vi "Index Created for lvproj.vi"(8 "error in (no error)":errorcluster, 11 "Indexing Test Finder Test in":refnum<class "Indexing Test Finder Test.lvclass">) -> (0 "error out":errorcluster, 3 "Indexing Test Finder Test out":refnum<class "Indexing Test Finder Test.lvclass">)   [LabVIEW 2020, in "LUnit Tests.lvlib" / "Indexing Test Finder Test.lvclass"]
uses:
  Indexing Test Finder Test.lvclass
  Indexing Test Finder Test.lvclass/Indexing Test Finder Test.ctl
  source/Framework/Helper Classes/Test Finder/Test Finder.lvclass
  Test Finder/Finder Test.lvclass
  c59a45e6-8387-4d73-9fe8-839093b27eb6.vi
  <vilib>/Astemes/LUnit/Test Case.lvclass
  C:/Git/astemes-lunit/tests/Test Finder/Finder Test.lvclass
  C:/Program Files (x86)/National Instruments/LabVIEW 2020/vi.lib/Astemes/LUnit/Test Case.lvclass
  C:/Git/astemes-lunit/tests/Indexing Test Finder Test/Indexing Test Finder Test.lvclass
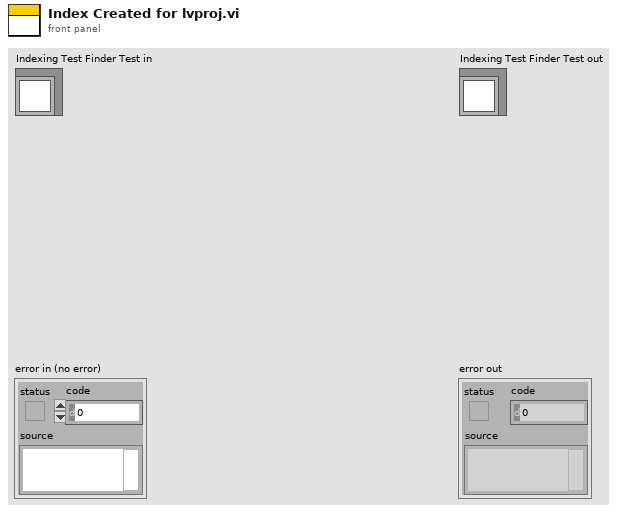
[diagram p1: front panel]
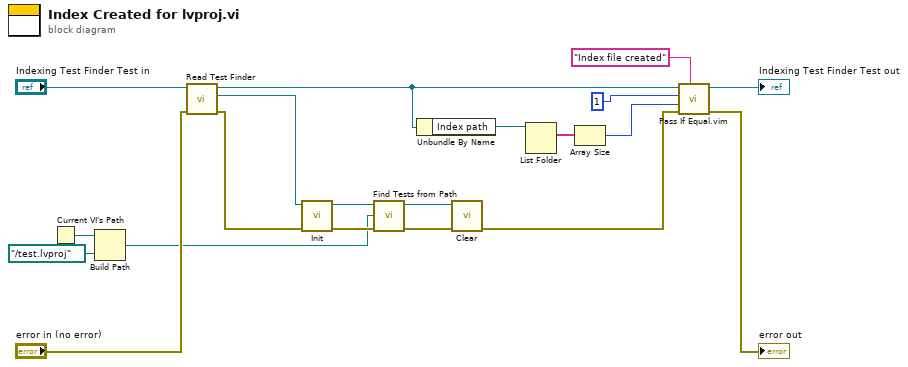
[diagram p0: block diagram]
diagram:
  n1 = Current VI's Path() -> (path=w12:path)
  n2 = Build Path(base path=w12, name or relative path=path "../test.lvproj") -> (appended path=w10:path)
  n3 = call "Read Test Finder.vi"("error in (no error)"="error in (no error)", "Test Finder In"="Indexing Test Finder Test in") -> ("error out"=w14:errorcluster, "Test Finder.lvclass"=w15:refnum<class "Test Finder.lvclass">, "Test Finder Out"=w4:refnum<class "Indexing Test Finder Test.lvclass">)  [unwired: 7 in]
  n4 = call-dynamic "Init.vi"("error in (no error)"=w14, "Test Finder in"=w15) -> ("error out"=w18:errorcluster, "Test Finder out"=w19:refnum<class "Test Finder.lvclass">)  [unwired: 8 in]
  n5 = call-dynamic "Find Tests from Path.vi"("error in (no error)"=w18, "Project or Class Path"=w10, "Test Case Finder In"=w19) -> ("error out"=w16:errorcluster, "Test Case Finder Out"=w17:refnum<class "Test Finder.lvclass">)  [unwired: 7 in]
  n6 = Unbundle By Name(w4) -> ("Index path"=w8:path)
  n7 = call "Clear.vi"("error in (no error)"=w16, "Test Finder in"=w17) -> ("error out"=w9:errorcluster)  [unwired: 8 in, 1 out]
  n8 = List Folder(path=w8) -> (filenames=w7:string[])  [unwired: 3 in, 3 out]
  n9 = Array Size(array=w7) -> (size(s)=w3:i32)
  n10 = call "Pass If Equal.vim"("Description"="Index file created", "error in (no error)"=w9, "Actual"=w3, "Expected"=1 ("size(s)"), "LUnit Test Case In"=w4) -> ("error out"=→"error out":errorcluster, "LUnit Test Case Out"=→"Indexing Test Finder Test out":refnum<class "Indexing Test Finder Test.lvclass">)  [unwired: 5 in]
